vi "test Parse Sorted Object Dictionary_4.vi"(11 "Test Case In":refnum<class "test Electronic Datasheet.lvclass">) -> (0 "error out":errorcluster, 3 "Test Case Out":refnum<class "test Electronic Datasheet.lvclass">)   [LabVIEW 2024, in "test Electronic Datasheet.lvclass"]
uses:
  test Electronic Datasheet.lvclass
  C:/Program Files/National Instruments/LabVIEW 2024/vi.lib/Astemes/LUnit/Test Case.lvclass
  Core/Object Type.ctl
  Core/Access Type.ctl
  <vilib>/Astemes/LUnit/Test Case.lvclass/Test Case.ctl
  <vilib>/Astemes/LUnit/Append Fail Result.vi
  <vilib>/Astemes/LUnit/Append Pass Result.vi
  <vilib>/Astemes/LUnit/Run In UI.vi
  <vilib>/Utility/error.llb/Clear Errors.vi
  Core/OD Sub-Entry/OD Sub-Entry.lvclass
  D:/git/EDS-File-Viewer/Core/OD Entry/OD Entry.lvclass
  Electronic Datasheet/utils/Electronic Datasheet_GetAttributes.vi
  Core/OD Entry/Get PDOMapping.vi
  Core/OD Entry/Get DefaultValue.vi
  Core/OD Entry/Get AccessType.vi
  Core/OD Entry/Get DataType.vi
  Core/OD Entry/Get ObjectType.vi
  Core/OD Entry/Get ParameterName.vi
  Electronic Datasheet/Electronic Datasheet.lvclass
  <vilib>/Astemes/LUnit/Test Case.lvclass
  Core/Electronic Datasheet.lvlib
  Core/OD Entry/OD Entry.lvclass
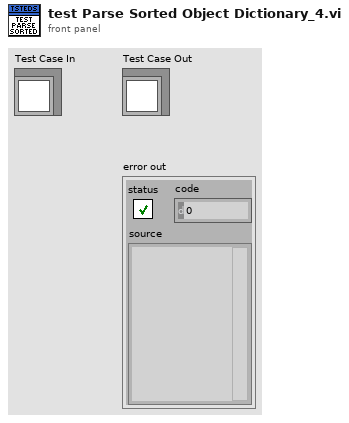
[diagram p1: front panel]
types:
  T1 = typedef "Electronic Datasheet.lvlib/Access Type.ctl" = enum16{"ro", "wo", "rw", "rwr", "rww", "const"}
  T2 = typedef "Electronic Datasheet.lvlib/Object Type.ctl" = u8
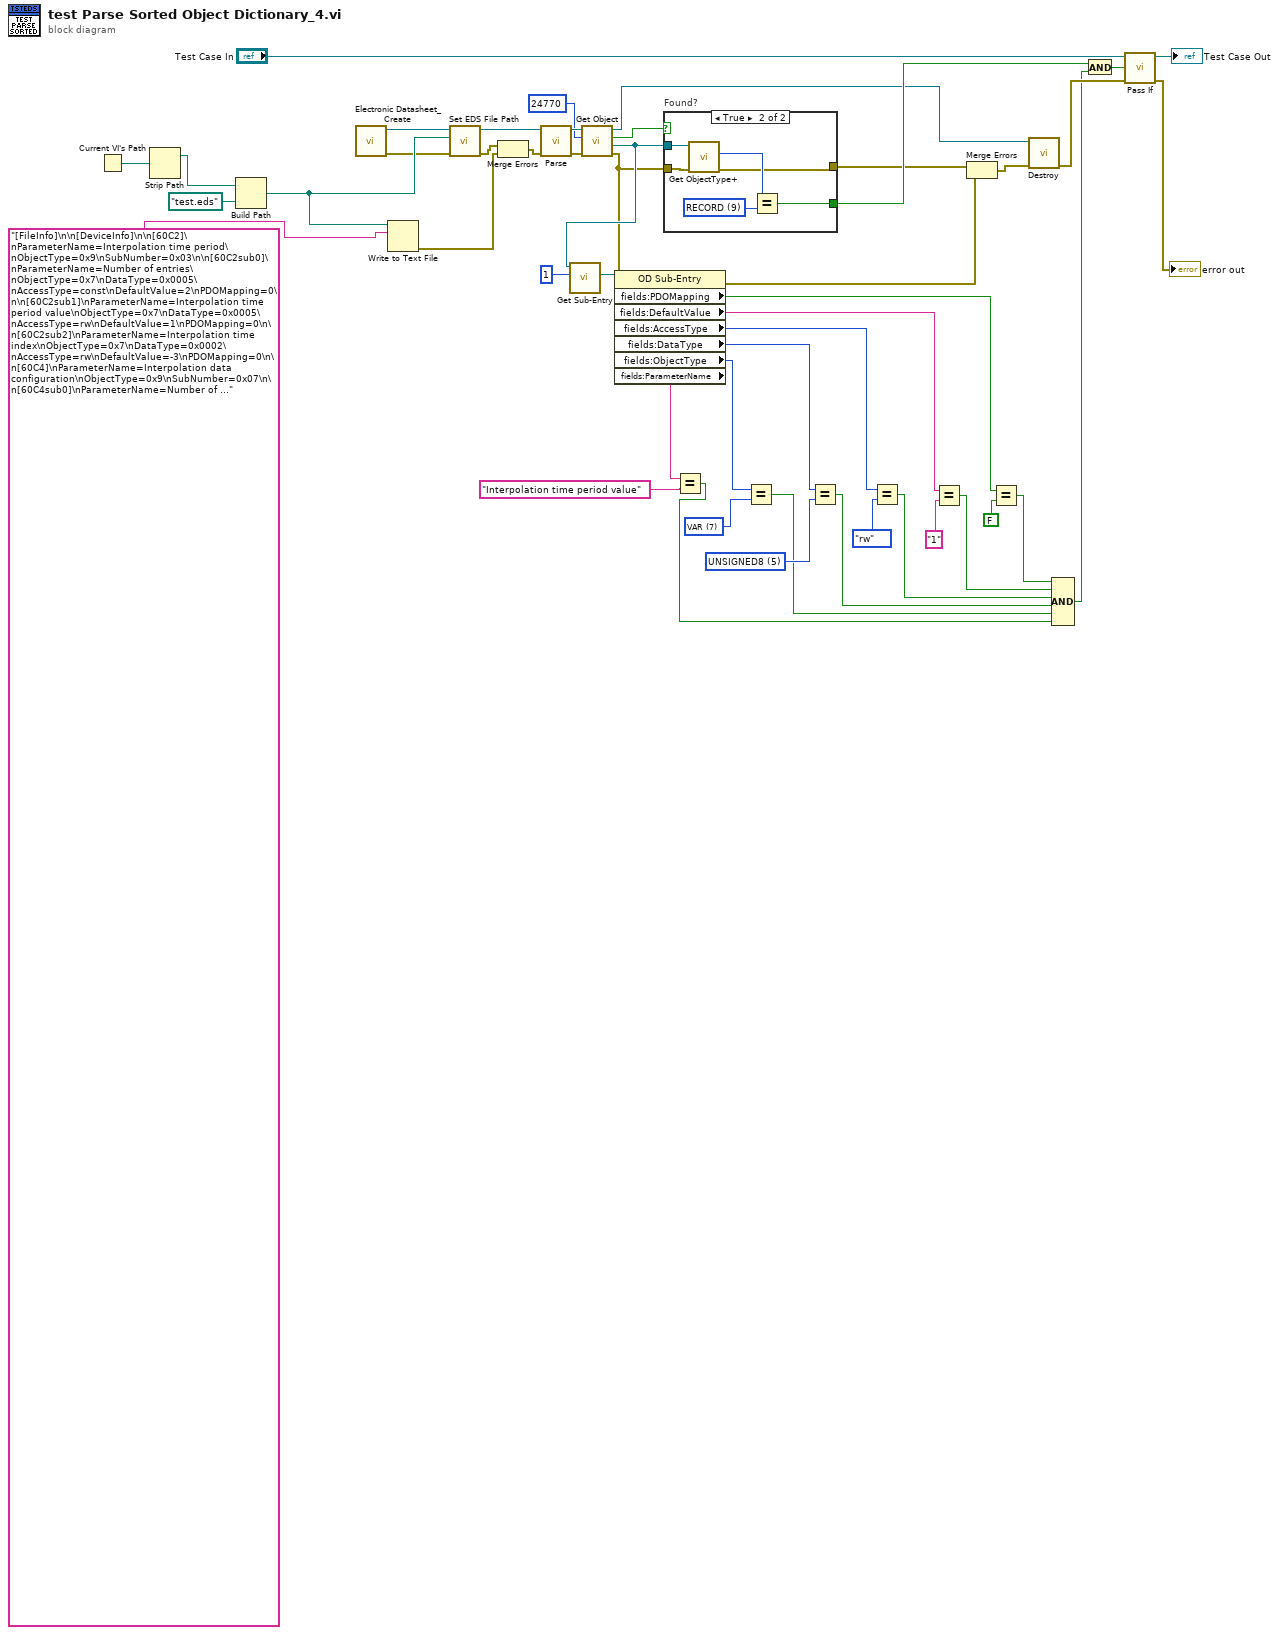
[diagram p0: block diagram]
diagram:
  w31 = u16 5 items=["BOOLEAN"=1, "INTEGER8"=2, "INTEGER16"=3, "INTEGER32"=4, "UNSIGNED8"=5, "UNSIGNED16"=6, "UNSIGNED32"=7, "REAL32"=8, "VISIBLE_STRING"=9, "OCTET_STRING"=10, "UNICODE_STRING"=11, "TIME_OF_DAY"=12, "TIME_DIFFERENCE"=13, "RESERVED1"=14, "DOMAIN"=15, "INTEGER24"=16, "REAL64"=17, "INTEGER40"=18, "INTEGER48"=19, "INTEGER56"=20, "INTEGER64"=21, "UNSIGNED24"=22, "RESERVED2"=23, "UNSIGNED40"=24, "UNSIGNED48"=25, "UNSIGNED56"=26, "UNSIGNED64"=27, "RESERVED3"=28, "RESERVED4"=29, "RESERVED5"=30, "RESERVED6"=31, "PDO_COMMUNICATION_PARAMETER"=32, "PDO_MAPPING"=33, "SDO_PARAMETER"=34, "IDENTITY"=35, "RESERVED7"=36] ("DataType")
  w32 = T2 7 items=["NULL"=0, "DOMAIN"=2, "DEFTYPE"=5, "DEFSTRUCT"=6, "VAR"=7, "ARRAY"=8, "RECORD"=9] ("ObjectType")
  n1 = Current VI's Path() -> (path=w44:path)
  n2 = Strip Path(path=w44) -> (stripped path=w40:path)  [unwired: 1 out]
  n3 = Build Path(base path=w40, name or relative path=path "test.eds") -> (appended path=w41:path)
  n4 = call "Electronic Datasheet_Create.vi"() -> ("Error Out"=w9:errorcluster, "reference out"=w10:refnum<class "Electronic Datasheet.lvclass">)  [unwired: 10 in]
  n5 = Write to Text File(file (use dialog)=w41, text="[FileInfo]\n\n[DeviceInfo]\n\n[60C2]\nParameterName=Interpolation time period\nObjectType=0x9\nSubNumber=0x03\n\n[60C2sub0]\nParameterName=Number of entries\nObjectType=0x7\nDataType=0x0005\nAccessType=const\nDefaultValue=2\nPDOMapping=0\n\n[60C2sub1]\nParameterName=Interpolation time period value\nObjectType=0x7\nDataType=0x0005\nAccessType=rw\nDefaultValue=1\nPDOMapping=0\n\n[60C2sub2]\nParameterName=Interpolation time index\nObjectType=0x7\nDataType=0x0002\nAccessType=rw\nDefaultValue=-3\nPDOMapping=0\n\n[60C4]\nParameterName=Interpolation data configuration\nObjectType=0x9\nSubNumber=0x07\n\n[60C4sub0]\nParameterName=Number of entries\nObjectType=0x7\nDataType=0x0005\nAccessType=const\nDefaultValue=6\nPDOMapping=0\n\n[60C4sub1]\nParameterName=MaximumBufferSize\nObjectType=0x7\nDataType=0x0007\nAccessType=ro\nDefaultValue=1\nPDOMapping=0\n\n[60C4sub2]\nParameterName=ActualBufferSize\nObjectType=0x7\nDataType=0x0007\nAccessType=rw\nDefaultValue=1\nPDOMapping=0\n\n[60C4sub3]\nParameterName=BufferOrganization\nObjectType=0x7\nDataType=0x0005\nAccessType=rw\nDefaultValue=0\nPDOMapping=0\n\n[60C4sub4]\nParameterName=BufferPosition\nObjectType=0x7\nDataType=0x0006\nAccessType=rw\nDefaultValue=1\nPDOMapping=0\n\n[60C4sub5]\nParameterName=SizeOfDataRecord\nObjectType=0x7\nDataType=0x0005\nAccessType=wo\nDefaultValue=4\nPDOMapping=0\n\n[60C4sub6]\nParameterName=BufferClear\nObjectType=0x7\nDataType=0x0005\nAccessType=wo\nDefaultValue=0\nPDOMapping=0") -> (error out=w42:errorcluster)  [unwired: 2 in, 2 out]
  n6 = call "Set EDS File Path.vi"("error in"=w9, "EDS File Path"=w41, "reference in"=w10) -> ("error out"=w1:errorcluster, "reference out"=w45:refnum<class "Electronic Datasheet.lvclass">)  [unwired: 7 in]
  n7 = Merge Errors(w1, w42) -> (w2:errorcluster)
  n8 = call "Parse.vi"("error in"=w2, "reference in"=w45) -> ("error out"=w8:errorcluster, "reference out"=w39:refnum<class "Electronic Datasheet.lvclass">)  [unwired: 8 in]
  n9 = call "Get Object.vi"("error in"=w8, "Index"=u16 24770 ("Numeric"), "reference in"=w39) -> ("error out"=w3:errorcluster, "OD Entry"=w5:refnum<class "OD Entry.lvclass">, "Found?"=w4:bool, "reference out"=w6:refnum<class "Electronic Datasheet.lvclass">)  [unwired: 5 in]
  n10 = call "Get Sub-Entry.vi"("Sub-Index"=u16 1, "reference in"=w5) -> ("OD Sub-Entry"=w18:refnum<class "OD Sub-Entry.lvclass">)  [unwired: 6 in, 3 out]
  n11 = property class="OD Sub-Entry"(reference=w18, error in=w3) -> (error out=w16:errorcluster, "fields:PDOMapping"=w17:bool, "fields:DefaultValue"=w15:string, "fields:AccessType"=w14:T1, "fields:DataType"=w13:u16, "fields:ObjectType"=w12:T2, "fields:ParameterName"=w11:string)  [unwired: 1 out]
  n12 = case "Found?" shown="True" w4 {
    selector: w4 -> [w49 _]
    tunnel: w5 -> [_ w56]
    tunnel: w3 -> [w50 w55]
    tunnel: [w49 w51] -> w37
    tunnel: [w50 w52] -> w35
    frame False {
    }
    frame True {
      w53 = T2 9 items=["NULL"=0, "DOMAIN"=2, "DEFTYPE"=5, "DEFSTRUCT"=6, "VAR"=7, "ARRAY"=8, "RECORD"=9] ("y")
      n13 = call "Get ObjectType+.vi"("Error In"=w55, "reference in"=w56) -> ("Error Out"=w52:errorcluster, "ObjectType"=w54:T2)  [unwired: 6 in, 2 out]
      n14 = Equal?(x=w54, y=w53) -> (x = y?=w51:bool)
    }
  }
  n15 = Equal?(x=w11, y="Interpolation time period value") -> (x = y?=w26:bool)
  n16 = Equal?(x=w12, y=w32) -> (x = y?=w25:bool)
  n17 = Equal?(x=w13, y=w31) -> (x = y?=w24:bool)
  n18 = Equal?(x=w14, y=Access_Type."rw") -> (x = y?=w23:bool)
  n19 = Equal?(x=w15, y="1") -> (x = y?=w22:bool)
  n20 = Merge Errors(w35, w16) -> (w20:errorcluster)
  n21 = Equal?(x=w17, y=FALSE) -> (x = y?=w21:bool)
  n22 = call-dynamic "Destroy.vi"("Error In"=w20, "reference in"=w6) -> ("Error Out"=w36:errorcluster)  [unwired: 8 in, 1 out]
  n23 = Compound Arithmetic op=AND(w21, w22, w23, w24, w25, w26) -> (w27:bool)
  n24 = And(x=w37, y=w27) -> (x .and. y?=w19:bool)
  n25 = call <vilib>:"Pass If.vi"("error in (no error)"=w36, "Pass?"=w19, "LUnit Test Case In"="Test Case In") -> ("error out"=→"error out":errorcluster, "LUnit Test Case Out"=→"Test Case Out":refnum<class "test Electronic Datasheet.lvclass">)  [unwired: 7 in]
